vi "macro_NumCmd_Send_Generic.vi"   [LabVIEW 2019, in "Trajectory_Library.lvlib"]
uses:
  VI/numCmd_ObtainQueue_Generic.vi
  Trajectory_Library.lvlib
  TypeDef/TRANSLATION3D.ctl
  TypeDef/QUATERNION.ctl
  TypeDef/ROTATION3D.ctl
  TypeDef/POSE3D.ctl
types:
  T1 = typedef "Trajectory_Library.lvlib/POSE3D.ctl" = cluster{"Translation3d":T2, "Rotation3d":T3}
  T2 = typedef "Trajectory_Library.lvlib/TRANSLATION3D.ctl" = cluster{"X":dbl, "Y":dbl, "Z":dbl}
  T3 = typedef "Trajectory_Library.lvlib/ROTATION3D.ctl" = cluster{"Q_quaternion":T4}
  T4 = typedef "Trajectory_Library.lvlib/QUATERNION.ctl" = cluster{"R":dbl, "V":dbl[]}
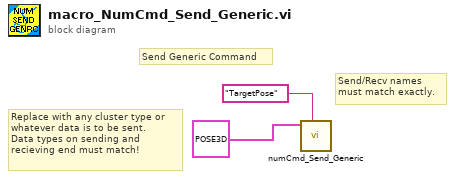
[diagram p0: block diagram]
diagram:
  # "Send/Recv names\nmust match exactly."
  # "Replace with any cluster type or \nwhatever data is to be sent.\nData types on sending and\nrecieving end must match!"
  # "Send Generic Command"
  n1 = call "numCmd_Send_Generic.vi"("Command Name"="TargetPose", "Value"=T1 {"Translation3d"={"X"=0.0, "Y"=0.0, "Z"=0.0}, "Rotation3d"={"Q_quaternion"={"R"=1.0, "V"=[0.0, 0.0, 0.0]}}} ("POSE3D")) -> ()  [unwired: 9 in, 1 out]
